vi "Stop Core.vi"(10 "final error code":i32, 11 "IED in":refnum<class "IED.lvclass">) -> (3 "IED out":refnum<class "IED.lvclass">)   [LabVIEW 2015, in "IED Actor.lvlib" / "IED.lvclass"]
doc: "(<B>Filename</B>: Actor Framework.lvlib:Actor.lvclass:Stop Core.vi)\n\nDefines what the actor does before it stops. Use the <B>final error code</B> input to determine whether the actor shut down in response to an error.\n\nBy default, this method does nothing. A descendant class may override it to define behavior, such as shutting down any processes the actor initiated in its override of the Actor Core method."
uses:
  IED.lvclass
  IED.lvclass/IED.ctl
  <vilib>/ActorFramework/Message Enqueuer/Message Enqueuer.lvclass/Message Enqueuer.ctl
  <vilib>/ActorFramework/Message Enqueuer/Enqueue.vi
  <vilib>/ActorFramework/Message Priority Queue/Priority Enqueue.vi
  <vilib>/ActorFramework/Actor/Actor.lvclass
  <vilib>/ActorFramework/Stop Msg/Stop Msg.lvclass
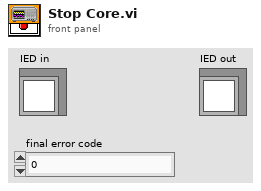
[diagram p1: front panel]
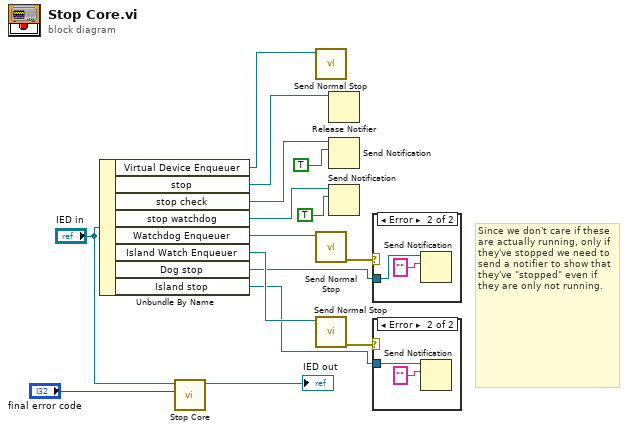
[diagram p0: block diagram]
diagram:
  # "Since we don't care if these are actually running, only if they've stopped we need to send a notifier to show that they've \"stopped\" even if they are only not running."
  n1 = Unbundle By Name("IED in") -> ("Virtual Device Enqueuer"=w1:refnum<class "Message Enqueuer.lvclass">, "stop"=w2:refnum<notifier>, "stop check"=w10:refnum<notifier>, "stop watchdog"=w9:refnum<notifier>, "Watchdog Enqueuer"=w8:refnum<class "Message Enqueuer.lvclass">, "Island Watch Enqueuer"=w7:refnum<class "Message Enqueuer.lvclass">, "Dog stop"=w5:refnum<notifier>, "Island stop"=w3:refnum<notifier>)
  n2 = call-parent "Stop Core.vi"("final error code"="final error code", "Actor in"="IED in") -> ("Actor out"=→"IED out":refnum<class "IED.lvclass">)  [unwired: 9 in]
  n3 = call <vilib>:"Send Normal Stop.vi"("Message Enqueuer"=w1) -> ()  [unwired: 10 in, 1 out]
  n4 = call <vilib>:"Send Normal Stop.vi"("Message Enqueuer"=w8) -> ("error out"=w6:errorcluster)  [unwired: 10 in]
  n5 = call <vilib>:"Send Normal Stop.vi"("Message Enqueuer"=w7) -> ("error out"=w4:errorcluster)  [unwired: 10 in]
  n6 = Release Notifier(notifier=w2) -> ()  [unwired: 2 in, 3 out]
  n7 = Send Notification(notification=TRUE, notifier=w10) -> ()  [unwired: 1 in, 2 out]
  n8 = Send Notification(notification=TRUE, notifier=w9) -> ()  [unwired: 1 in, 2 out]
  n9 = case shown="Error" w6 {
    tunnel: w5 -> [_ w17]
    frame No Error {
    }
    frame Error {
      n10 = Send Notification(notification="", notifier=w17) -> ()  [unwired: 1 in, 2 out]
    }
  }
  n11 = case shown="Error" w4 {
    tunnel: w3 -> [_ w19]
    frame No Error {
    }
    frame Error {
      n12 = Send Notification(notification="", notifier=w19) -> ()  [unwired: 1 in, 2 out]
    }
  }
